vi "Timer Action Engine.vi"(9 "Current State":bool, 10 "Time Duration (s)":dbl, 11 "Action":T1) -> (0 "Quit Timer":bool, 1 "Clock Output":bool, 2 "Pulse Out":bool, 3 "Time Elapsed":dbl)   [LabVIEW 2021]
uses:
  Controls/Timer Actions.ctl
panel:
  # "Momentary Pulse O/P"
  # "Square Wave Pulse O/P"
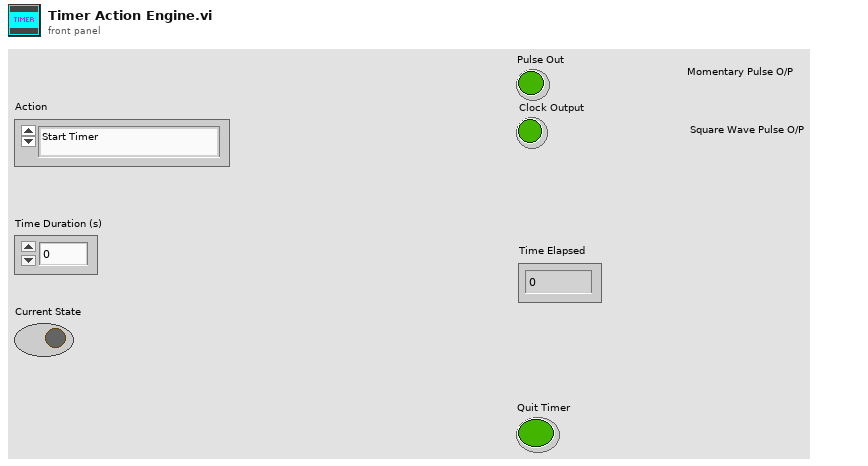
[diagram p1: front panel]
types:
  T1 = typedef "Timer Actions.ctl" = enum16{"Start Timer", "Restart Timer", "Check Timer", "Pause Timer", "Reset Timer", "Exit Timer"}
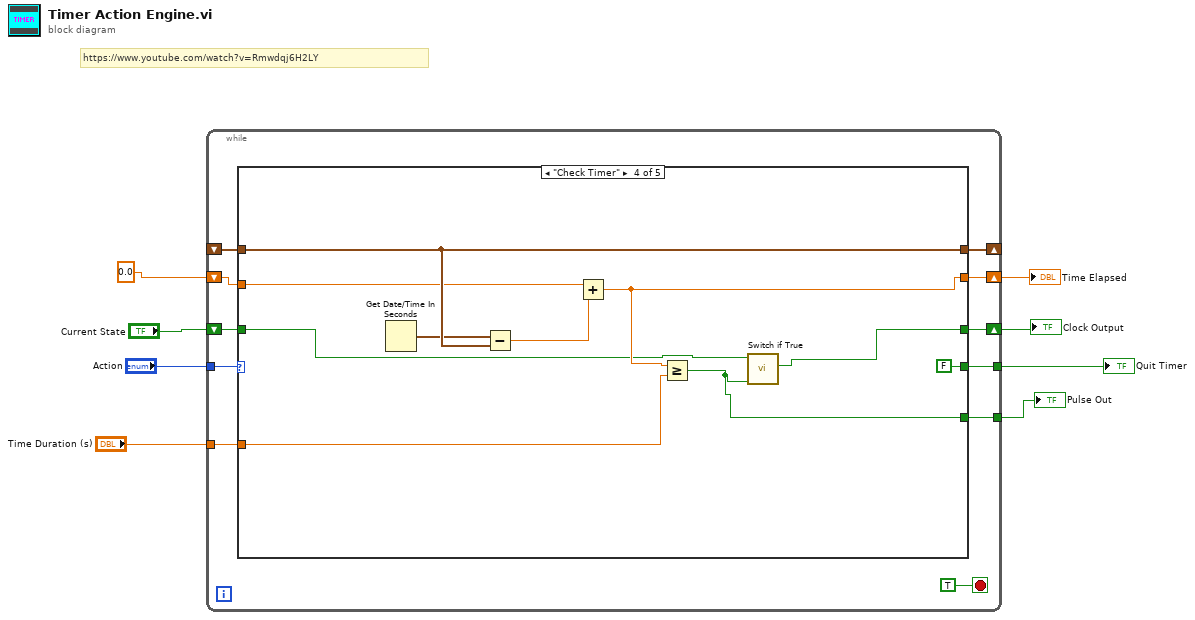
[diagram p0: block diagram]
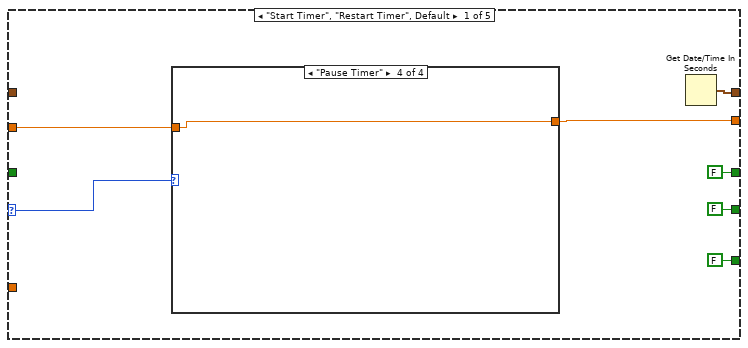
[diagram p2: hidden frame]
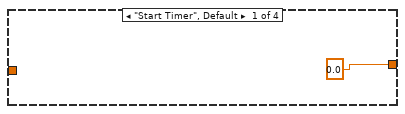
[diagram p3: hidden frame]
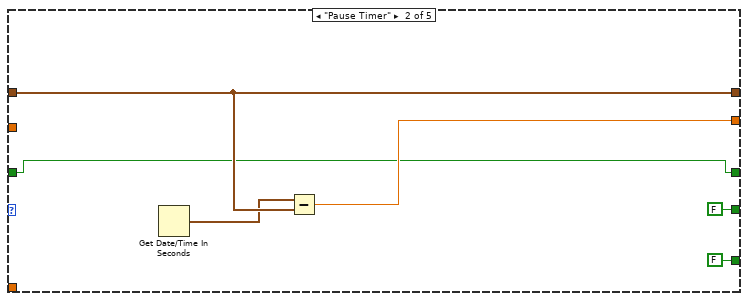
[diagram p6: hidden frame]
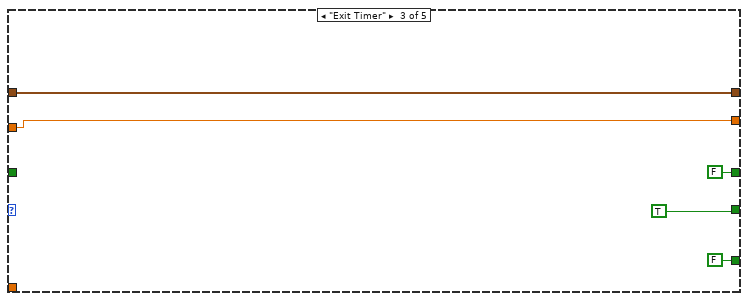
[diagram p7: hidden frame]
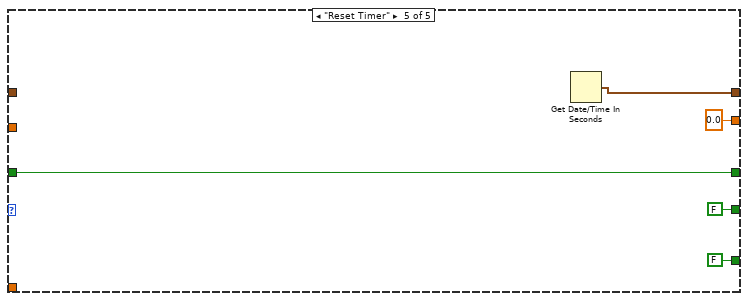
[diagram p8: hidden frame]
diagram:
  # "https://www.youtube.com/watch?v=Rmwdqj6H2LY"
  n1 = while {
    tunnel: "Action" -> [w19]
    shift-right: [w18] -> _
    shift-left: _ -> [w14]
    shift-right: [w17] -> w6
    shift-left: 0.0 ("Time Elapsed") -> [w15]
    tunnel: "Time Duration (s)" -> [w13]
    tunnel: [w12] -> w4
    shift-right: [w11] -> w3
    shift-left: "Current State" -> [w10]
    tunnel: [w9] -> w2
    stop <- TRUE stop-if-true
    n2 = case shown="\"Check Timer\"" w19 {
      selector: w19 -> [w25 _ _ _ _]
      tunnel: [w26 w36 w41 w51 w54] -> w18
      tunnel: [w24 w34 w40 w47 0.0 ("Time Elapsed")] -> w17
      tunnel: w15 -> [w23 _ w40 w48 _]
      tunnel: w14 -> [_ w36 w41 w51 _]
      tunnel: w13 -> [_ _ _ w46 _]
      tunnel: [FALSE FALSE TRUE FALSE FALSE] -> w12
      tunnel: [FALSE w31 FALSE w43 w53] -> w11
      tunnel: w10 -> [_ w31 _ w44 w53]
      tunnel: [FALSE FALSE FALSE w42 FALSE] -> w9
      frame "Start Timer", "Restart Timer", Default {
        n3 = case shown="\"Pause Timer\"" w25 {
          tunnel: [0.0 ("Time Elapsed") w28 w29 w30] -> w24
          tunnel: w23 -> [_ w28 w29 w30]
          frame "Start Timer", Default {
          }
          frame "Restart Timer" {
          }
          frame "Check Timer" {
          }
          frame "Pause Timer" {
          }
        }
        n4 = Get Date/Time In Seconds() -> (seconds since 1Jan1904=w26:timestamp)
      }
      frame "Pause Timer" {
        n5 = Get Date/Time In Seconds() -> (seconds since 1Jan1904=w35:timestamp)
        n6 = Subtract(x=w35, y=w36) -> (x-y=w34:dbl)
      }
      frame "Exit Timer" {
      }
      frame "Check Timer" {
        n7 = Get Date/Time In Seconds() -> (seconds since 1Jan1904=w50:timestamp)
        n8 = Subtract(x=w50, y=w51) -> (x-y=w49:dbl)
        n9 = Add(x=w48, y=w49) -> (x+y=w47:dbl)
        n10 = Greater Or Equal?(x=w47, y=w46) -> (x >= y?=w42:bool)
        n11 = call "Switch if True.vi"("Switch State"=w42, "Current State"=w44) -> ("State Out"=w43:bool)  [unwired: 9 in]
      }
      frame "Reset Timer" {
        n12 = Get Date/Time In Seconds() -> (seconds since 1Jan1904=w54:timestamp)
      }
    }
  }
  "Quit Timer" <- w4
  "Time Elapsed" <- w6
  "Clock Output" <- w3
  "Pulse Out" <- w2
